vi "Form Response Log Text.vi"(6 "ACK":bool, 8 "error in":errorcluster, 10 "Ack Data Input":string, 11 "Module Action":string) -> (3 "String to Write":string)   [LabVIEW 2015, in "Generic Module Library.lvlib" / "Template G_Module.lvlib"]
uses:
  Template G_Module.lvlib
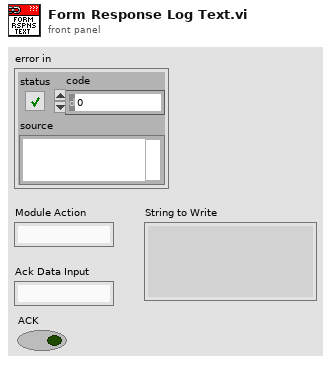
[diagram p1: front panel]
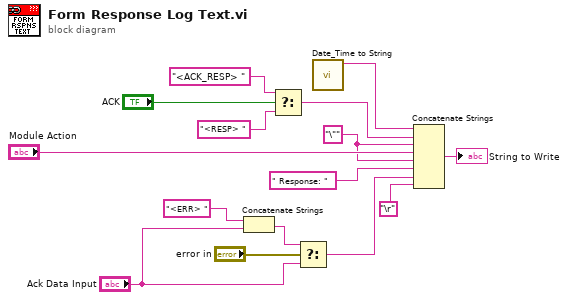
[diagram p0: block diagram]
diagram:
  w10 = "\"" ("string")
  n1 = Concatenate Strings("<ERR> " ("string"), "Ack Data Input") -> (w4:string)
  n2 = Select(t="<ACK_RESP> " ("string"), s="ACK", f="<RESP> " ("string")) -> (s? t:f=w8:string)
  n3 = Select(t=w4, s="error in", f="Ack Data Input") -> (s? t:f=w1:string)
  n4 = call "Date_Time to String.vi"() -> ("date/time string"=w14:string)  [unwired: 11 in]
  n5 = Concatenate Strings(w14, w8, w10, "Module Action", w10, " Response: " ("string"), w1, "\r") -> (→"String to Write":string)
